vi "GetIniScripts.vi"(7 "section":string="Script", 8 "ErrorArray":errorcluster[](array[cluster]), 10 "ModuleNameArray":string[](array[string]), 11 "Test.lvclass":refnum<class "Test.lvclass">) -> (0 "ErrorArray":errorcluster[](array[cluster]), 2 "Script":string[](array[string]), 3 "Test.lvclass":refnum<class "Test.lvclass">)   [LabVIEW 2018, in "Test.lvclass"]
uses:
  Test.lvclass
  Test.lvclass/Test.ctl
  Accessors/Read ErrorSeverity.vi
  Accessors/Read PluginPathArray.vi
  Accessors/Read PluginIndex.vi
  <vilib>/Utility/error.llb/Error Cluster From Error Code.vi
  <vilib>/ErrorRing/Error Ring.xnode
  <vilib>/Utility/config.llb/NI_LVConfig.lvlib
  <userlib>/NIST/NISTErrorLib/NISTErrorLib.lvlib
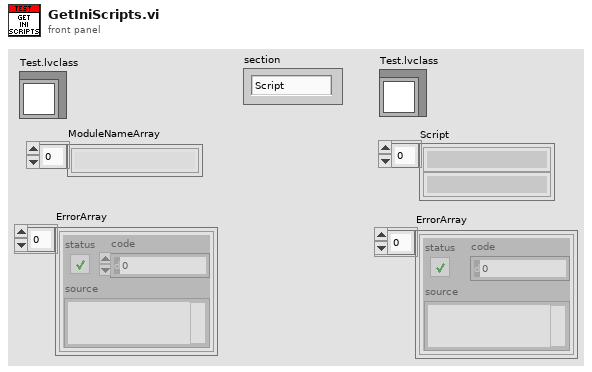
[diagram p1: front panel]
types:
  T1 = typedef "NI_LVConfig.lvlib/Config Data RefNum.ctl" = refnum<k1>
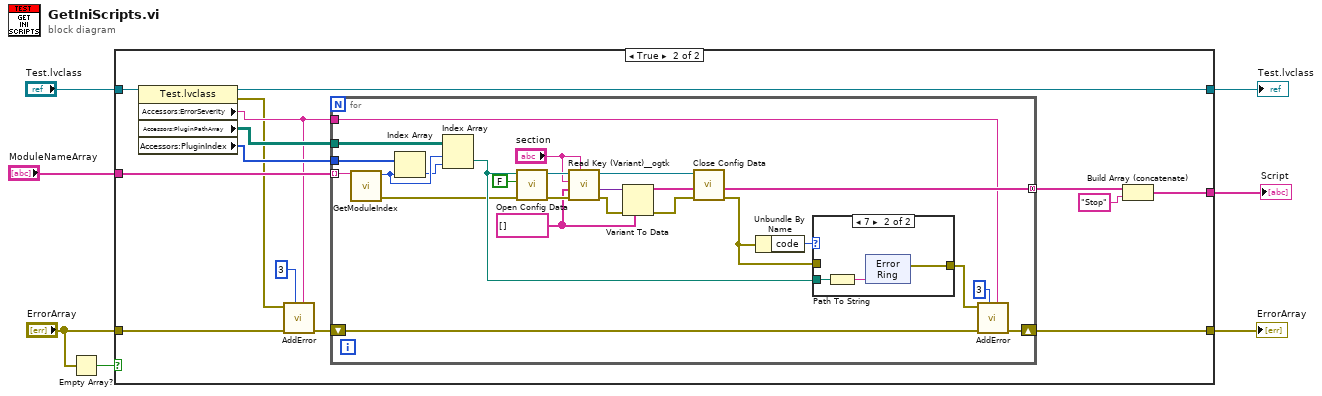
[diagram p0: block diagram]
diagram:
  n1 = Empty Array?(array="ErrorArray") -> (empty?=w7:bool)
  n2 = case shown="True" w7 {
    tunnel: "ErrorArray" -> [w8 w12]
    tunnel: "Test.lvclass" -> [w9 w23]
    tunnel: [w9 w21] -> w4
    tunnel: [w8 w17] -> w3
    tunnel: "ModuleNameArray" -> [_ w22]
    tunnel: [_ w16] -> w1
    frame False {
    }
    frame True {
      n3 = property class="Test.lvclass"(reference=w23) -> (reference out=w21:refnum<class "Test.lvclass">, error out=w13:errorcluster, "Accessors:ErrorSeverity"=w14:string, "Accessors:PluginPathArray"=w19:path[][], "Accessors:PluginIndex"=w20:u32[])  [unwired: 1 in]
      n4 = call <userlib>:"AddError.vi"("Severity"=w14, "Priority"=u8 3, "ErrorArray"=w12, "error in (no error)"=w13) -> ("ErrorArray"=w11:errorcluster[])  [unwired: 6 in, 1 out]
      n5 = for {
        tunnel: w22 -> [w30] mode=indexing
        tunnel: w20 -> [w47]
        tunnel: w19 -> [w46]
        tunnel: [w37] -> w18 mode=concatenating
        shift-right: [w36] -> w17
        shift-left: w11 -> [w35]
        tunnel: w14 -> [w33]
        w39 = string[] []
        n6 = call "GetModuleIndex.vi"("ModuleType"=w30) -> ("ModuleIndex"=w28:i32, "Error"=w29:errorcluster)  [unwired: 9 in]
        n7 = Index Array(array=w47, index=w28) -> (element=w27:u32)
        n8 = Index Array(array=w46, index (row)=w28, index (col)=w27) -> (element=w31:path)
        n9 = call <vilib>:"Open Config Data.vi"("error in (no error)"=w29, "create file if necessary (T)"=FALSE, "configuration file path"=w31) -> ("error out"=w42:errorcluster, "refnum"=w44:T1)  [unwired: 6 in, 1 out]
        n10 = call <userlib>:"Read Key (Variant)__ogtk.vi"("section"="section", "error in (no error)"=w42, "type"=w39, "key (optional)"="section", "refnum"=w44) -> ("error out"=w40:errorcluster, "key-value"=w41:variant, "refnum out"=w26:T1)  [unwired: 3 in, 1 out]
        n11 = Variant To Data(error in=w40, type=w39, Variant=w41) -> (data=w37:string[], error out=w25:errorcluster)
        n12 = call <vilib>:"Close Config Data.vi"("error in (no error)"=w25, "refnum"=w26) -> ("error out"=w24:errorcluster)  [unwired: 8 in, 1 out]
        n13 = Unbundle By Name(w24) -> ("code"=w38:i32)
        n14 = case shown="7" w38 {
          tunnel: w24 -> [w48 _]
          tunnel: [w48 w51] -> w34
          tunnel: w31 -> [_ w50]
          frame 0, Default {
          }
          frame 7 {
            n15 = Path To String(path=w50) -> (string=w49:string)
            n16 = xnode "Error Ring"("parameter 0"=w49) -> ("error out"=w51:errorcluster)
          }
        }
        n17 = call <userlib>:"AddError.vi"("Severity"=w33, "Priority"=u8 3, "ErrorArray"=w35, "error in (no error)"=w34) -> ("ErrorArray"=w36:errorcluster[])  [unwired: 6 in, 1 out]
      }
      n18 = Build Array (concatenate)(w18, "Stop") -> (w16:string[])
    }
  }
  "Test.lvclass" <- w4
  "ErrorArray" <- w3
  "Script" <- w1
